vi "PH_gentec_P-Link.Action get Info.vi"(0 "i ref in":refnum<vi>, 5 "error in":errorcluster) -> (14 "i ref out":refnum<vi>, 19 "error out":errorcluster)   [LabVIEW 2014, in "PH_gentec_P-Link.lvlib"]
doc: "This VI gets the basic information from the device."
uses:
  PH_gentec_P-Link.lvlib
  instr.lib/Gentec-M-Link/Driver/Type Defs/gentec-M-Link.Range.ctl
  PH_Basics/PH_Powermeter_BaseClass/PH_Powermeter_BaseClass.State.ctl
  PH_Basics/PH_Powermeter_BaseClass/PH_Powermeter_BaseClass.Head Attributes.ctl
  PH_Basics/PH_Powermeter_BaseClass/PH_gentec_BaseClass.Head Settings.ctl
  PH_Basics/PH_Powermeter_BaseClass/PH_Powermeter_BaseClass.lvlib
  instr.lib/Gentec-P-Link/gentec-P-Link - Driver.lvlib
  instr.lib/Gentec-M-Link/gentec-M-Link - Driver.lvlib
panel:
  in  "Dummy":T1 items=["1f", "3f", "10f", "30f", "100f", "300f", "1p", "3p", "10p", "30p", "100p", "300p", "1n", "3n", "10n", "30n", "100n", "300n", "1u", "3u", "10u", "30u", "100u", "300u", "1m", "3m", "10m", "30m", "100m", "300m", "1", "3", "10", "30", "100", "300", "1K", "3K", "10K", "30K", "100K", "300K", "1M", "3M", "10M", "30M", "100M", "300M"]
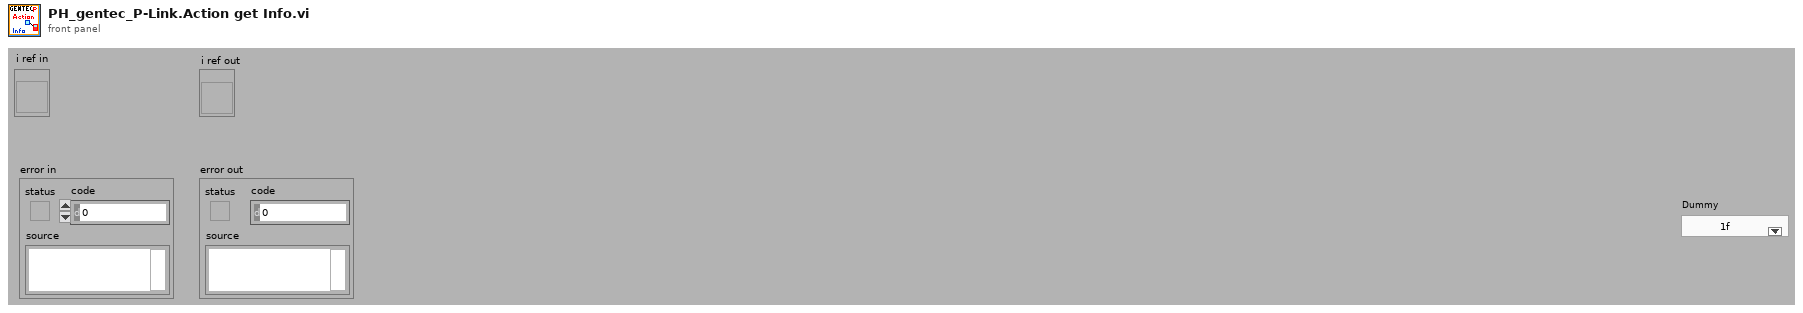
[diagram p1: front panel]
types:
  T1 = typedef "gentec-M-Link - Driver.lvlib/gentec-M-Link.Range.ctl" = u16
  T2 = typedef "PH_Powermeter_BaseClass.lvlib/PH_gentec_BaseClass.Head Settings.ctl" = cluster{"Trigger Level":dbl, "Wavelength":u32, "Range":u32}
  T3 = typedef "PH_Powermeter_BaseClass.lvlib/PH_Powermeter_BaseClass.Head Attributes.ctl" = cluster{"Instrument Type":string, "Head Version":string, "Head Name":string, "Serial Number":string, "Firmware":string, "Sensor Type":string, "MinimumRange":u32, "Maximum Range":u32, "Min Wavelength":i32, "Max Wavelength":i32}
  T4 = typedef "PH_Powermeter_BaseClass.lvlib/PH_Powermeter_BaseClass.State.ctl" = enum32{"off", "operating", "opened", "checked", "connected", "Sets to change", "running"}
  T5 = typedef "PH_Powermeter_BaseClass.lvlib/PH_Powermeter_BaseClass.i attribute.ctl" = cluster{"GUI References":T6, "Connection":T7, "Head Attributes":T3, "VISA resource":refnum<visa-resource-name>, "Energy":T8, "Service ID Energy":i32, "Wanted Settings":T2, "Current Settings":T2}
  T6 = typedef "PH_Powermeter_BaseClass.lvlib/PH_Powermeter_BaseClass.GUI Refs.ctl" = cluster{"Head Attributes":refnum<vi>, "Energy":refnum<vi>, "Connection":refnum<vi>, "VISA Resource":refnum<vi>, "Scaling Factor":refnum<vi>, "Range":refnum<vi>, "Wavelength":refnum<vi>, "Trigger Level":refnum<vi>, "Wanted Settings":refnum<vi>, "Current Settings":refnum<vi>}
  T7 = typedef "PH_Powermeter_BaseClass.lvlib/PH_Powermeter_BaseClass.Connection.ctl" = cluster{"failed checks":i8, "Timeout":bool, "Data read":string, "Failure":bool, "Error":bool, "State":T4}
  T8 = typedef "PH_Powermeter_BaseClass.lvlib/PH_Powermeter_BaseClass.Energy.ctl" = cluster{"current Value":dbl, "unscaled":dbl, "Scaling Factor":dbl}
  T9 = typedef "LVStringsAndValuesArrayTypeDef_U16.ctl" = cluster{"String":string, "Value":u16}[]
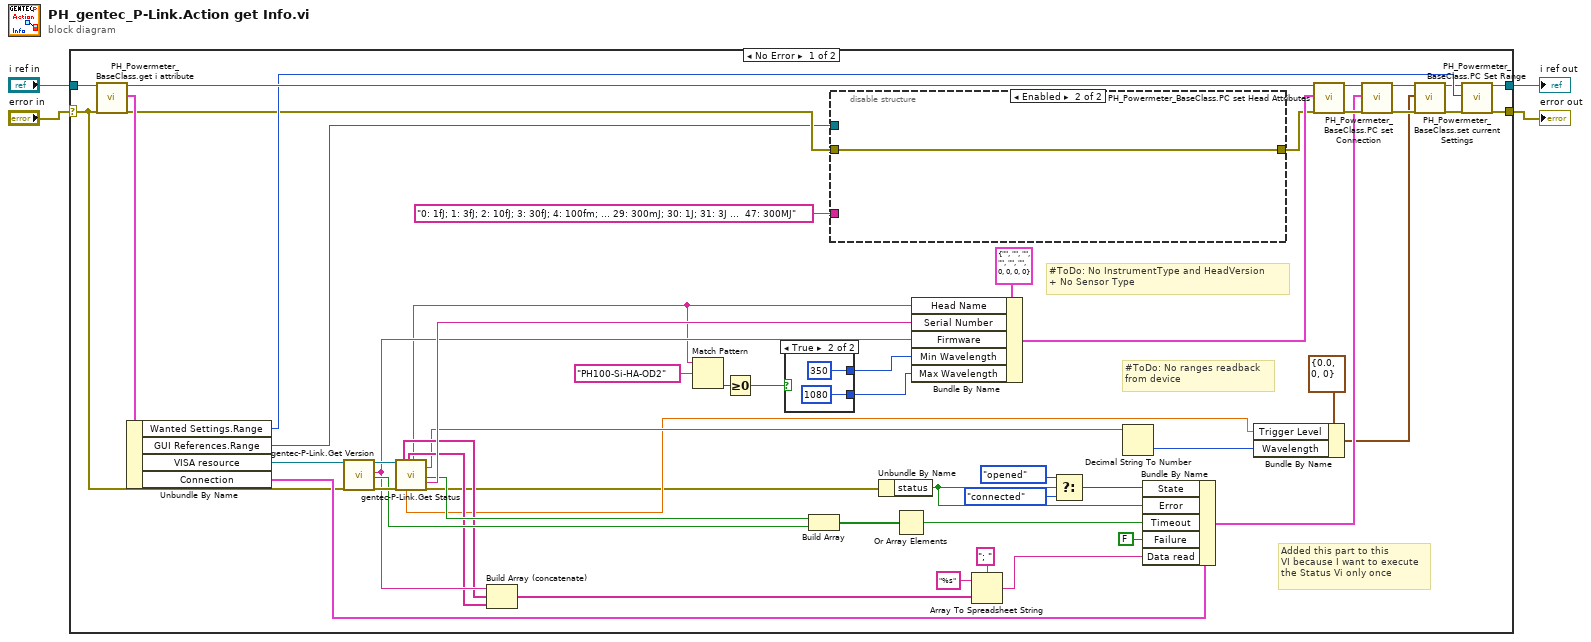
[diagram p0: block diagram]
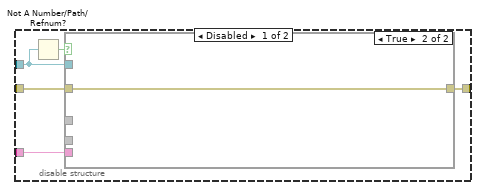
[diagram p3: hidden frame]
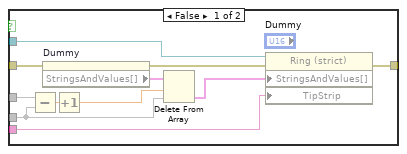
[diagram p4: hidden frame]
diagram:
  n1 = case shown="No Error" "error in" {
    selector: "error in" -> [w28 w79]
    tunnel: [w38 w79] -> w3
    tunnel: "i ref in" -> [w47 w78]
    tunnel: [w37 w78] -> w1
    frame No Error {
      # "Added this part to this\nVI because I want to execute\nthe Status Vi only once"
      # "#ToDo: No ranges readback\nfrom device"
      # "#ToDo: No InstrumentType and HeadVersion\n+ No Sensor Type"
      n2 = call "PH_Powermeter_BaseClass.get i attribute.vi"("i ref in"=w47, "error in (no error)"=w28) -> ("i ref out"=w46:refnum<vi>, "i attribute"=w42:T5, "error out"=w35:errorcluster)  [unwired: 15 in]
      n3 = Unbundle By Name(w42) -> ("Wanted Settings.Range"=w36:u32, "GUI References.Range"=w33:refnum<vi>, "VISA resource"=w29:refnum<visa-resource-name>, "Connection"=w41:T7)
      n4 = call "gentec-P-Link.Get Version.vi"("VISA resource name"=w29, "error in (no error)"=w28) -> ("VISA resource name"=w30:refnum<visa-resource-name>, "Version"=w24:string, "TimeOut?"=w25:bool, "error out"=w31:errorcluster)  [unwired: 14 in]
      n5 = call "gentec-P-Link.Get Status.vi"("VISA resource name"=w30, "error in (no error)"=w31) -> ("Status1"=w23:string[], "Status2"=w22:string[], "TriggerLevel"=w13:dbl, "Head Model Name"=w10:string, "Wavelength"=w16:string, "TimeOut?"=w26:bool, "Head S/N"=w27:string, "error out"=w12:errorcluster)  [unwired: 5 in, 5 out]
      n6 = Build Array (concatenate)(w24, w23, w22) -> (w55:string[])
      n7 = Match Pattern(string=w10, regular expression="PH100-Si-HA-OD2" ("y")) -> (offset past match=w8:i32)  [unwired: 1 in, 3 out]
      n8 = Greater Or Equal To 0?(x=w8) -> (x >= 0?=w7:bool)
      n9 = case shown="True" w7 {
        tunnel: [_ 350 ("Min Wavelength")] -> w6
        tunnel: [_ 1080 ("Min Wavelength")] -> w5
        frame False {
        }
        frame True {
        }
      }
      n10 = Build Array(w26, w25) -> (w57:bool[])
      n11 = disable-structure shown="Enabled" {
        disable-tunnel: w35 -> [w64 w77]
        disable-tunnel: [w63 w77] -> w34
        disable-tunnel: w33 -> [w61 _]
        disable-tunnel: "0: 1fJ; 1: 3fJ; 2: 10fJ; 3: 30fJ; 4: 100fm; ... 29: 300mJ; 30: 1J; 31: 3J ...  47: 300MJ" -> [w60 _]
        frame Disabled {
          n12 = Not A Number/Path/Refnum?(number/path/refnum=w61) -> (NaN/Path/Refnum?=w62:bool)
          n13 = case shown="True" w62 {
            tunnel: [w75 w76] -> w63
            tunnel: w61 -> [w74 _]
            tunnel: w64 -> [w73 w76]
            tunnel: _ -> [w67 _]
            tunnel: _ -> [w70 _]
            tunnel: w60 -> [w65 _]
            frame False {
              n14 = Subtract(x=w70, y=w67) -> (x-y=w69:dbl)
              n15 = property on="Dummy" class="Ring (strict)"(error in=w73) -> (error out=w72:errorcluster, "StringsAndValues[]"=w71:T9)  [unwired: 1 in, 1 out]
              n16 = Increment(x=w69) -> (x+1=w68:dbl)
              n17 = Delete From Array(array=w71, length=w68, index=w67) -> (deleted portion=w66:T9)  [unwired: 1 out]
              n18 = property class="Ring (strict)"(reference=w74, error in=w72, "StringsAndValues[]"=w66, "TipStrip"=w65) -> (error out=w75:errorcluster)  [unwired: 1 out]
            }
            frame True {
            }
          }
        }
        frame Enabled {
        }
      }
      n19 = Unbundle By Name(w12) -> ("status"=w51:bool)
      n20 = Or Array Elements(Boolean array=w57) -> (logical OR=w56:bool)
      n21 = Bundle By Name(cluster=T3 {"Instrument Type"="", "Head Version"="", "Head Name"="", "Serial Number"="", "Firmware"="", "Sensor Type"="", "MinimumRange"=0, "Maximum Range"=0, "Min Wavelength"=0, "Max Wavelength"=0} ("Head Attributes"), "Head Name"=w10, "Serial Number"=w27, "Firmware"=w24, "Min Wavelength"=w6, "Max Wavelength"=w5) -> (w39:T3)
      n22 = Array To Spreadsheet String(delimiter (Tab)="; ", array=w55, 3:"%s" ("format string")) -> (spreadsheet string=w52:string)
      n23 = Select(t=PH_Powermeter_BaseClass.State."opened" ("State"), s=w51, f=PH_Powermeter_BaseClass.State."connected") -> (s? t:f=w49:T4)
      n24 = Decimal String To Number(string=w16) -> (number=w15:i32)  [unwired: 2 in, 1 out]
      n25 = Bundle By Name(cluster=w41, "State"=w49, "Error"=w51, "Timeout"=w56, "Failure"=FALSE, "Data read"=w52) -> (w43:T7)
      n26 = Bundle By Name(cluster=T2 {"Trigger Level"=0.0, "Wavelength"=0, "Range"=0} ("Current Settings"), "Trigger Level"=w13, "Wavelength"=w15) -> (w14:T2)
      n27 = call "PH_Powermeter_BaseClass.PC set Head Attributes.vi"("VI in"=w46, "Head Attributes"=w39, "error in (no error)"=w34) -> ("VI out"=w45:refnum<vi>, "error out"=w44:errorcluster)  [unwired: 15 in]
      n28 = call "PH_Powermeter_BaseClass.PC set Connection.vi"("VI in"=w45, "Connection"=w43, "error in (no error)"=w44) -> ("VI out"=w18:refnum<vi>, "error out"=w21:errorcluster)  [unwired: 15 in]
      n29 = call "PH_Powermeter_BaseClass.set current Settings.vi"("VI in"=w18, "Current Settings"=w14, "error in (no error)"=w21) -> ("VI out"=w19:refnum<vi>, "error out"=w20:errorcluster)  [unwired: 15 in]
      n30 = call "PH_Powermeter_BaseClass.PC Set Range.vi"("VI in"=w19, "Wanted Range"=w36, "error in (no error)"=w20) -> ("VI out"=w37:refnum<vi>, "error out"=w38:errorcluster)  [unwired: 15 in]
    }
    frame Error {
    }
  }
  "error out" <- w3
  "i ref out" <- w1
